vi "Drive_Strait.vi"(8 "Right MotorControlDevRef in":T1={"DeviceStatus"={"status"=FALSE, "code"=0, "source"=""}, "Type"=enum."PWM", "PWM"={"PWM Channel"=enum."Invalid", "DeadBand"={"Name"="", "maxPositivePwm"=0, "minPositivePwm"=0, "centerPwm"=0, "maxNegativePwm"=0, "minNegativePwm"=0, "angularRange"=0}}, "CAN"={"Device Number"=0, "SetOutput VI Ref"=variant(refnum<vi> refnum), "GetOutput VI Ref"=variant(refnum<vi> refnum), "Enable VI Ref"=variant(refnum<vi> refnum), "Disable VI Ref"=variant(refnum<vi> refnum), "Data"=variant}, "Invert"=FALSE}, 9 "Left MotorControlDevRef in":T1={"DeviceStatus"={"status"=FALSE, "code"=0, "source"=""}, "Type"=enum."PWM", "PWM"={"PWM Channel"=enum."Invalid", "DeadBand"={"Name"="", "maxPositivePwm"=0, "minPositivePwm"=0, "centerPwm"=0, "maxNegativePwm"=0, "minNegativePwm"=0, "angularRange"=0}}, "CAN"={"Device Number"=0, "SetOutput VI Ref"=variant(refnum<vi> refnum), "GetOutput VI Ref"=variant(refnum<vi> refnum), "Enable VI Ref"=variant(refnum<vi> refnum), "Disable VI Ref"=variant(refnum<vi> refnum), "Data"=variant}, "Invert"=FALSE}, 11 "Distance in":dbl format="%#_13g") -> (0 "Right MotorControlDevRef out":T1={"DeviceStatus"={"status"=FALSE, "code"=0, "source"=""}, "Type"=enum."PWM", "PWM"={"PWM Channel"=enum."Invalid", "DeadBand"={"Name"="", "maxPositivePwm"=0, "minPositivePwm"=0, "centerPwm"=0, "maxNegativePwm"=0, "minNegativePwm"=0, "angularRange"=0}}, "CAN"={"Device Number"=0, "SetOutput VI Ref"=variant(refnum<vi> refnum), "GetOutput VI Ref"=variant(refnum<vi> refnum), "Enable VI Ref"=variant(refnum<vi> refnum), "Disable VI Ref"=variant(refnum<vi> refnum), "Data"=variant}, "Invert"=FALSE}, 1 "Left MotorControlDevRef out":T1={"DeviceStatus"={"status"=FALSE, "code"=0, "source"=""}, "Type"=enum."PWM", "PWM"={"PWM Channel"=enum."Invalid", "DeadBand"={"Name"="", "maxPositivePwm"=0, "minPositivePwm"=0, "centerPwm"=0, "maxNegativePwm"=0, "minNegativePwm"=0, "angularRange"=0}}, "CAN"={"Device Number"=0, "SetOutput VI Ref"=variant(refnum<vi> refnum), "GetOutput VI Ref"=variant(refnum<vi> refnum), "Enable VI Ref"=variant(refnum<vi> refnum), "Disable VI Ref"=variant(refnum<vi> refnum), "Data"=variant}, "Invert"=FALSE}, 3 "Drive time out":u32)   [LabVIEW 2016]
uses:
  <vilib>/Rock Robotics/WPI/MotorControl/WPI_MotorControlDeviceRef.ctl
  <vilib>/Rock Robotics/WPI/MotorControl/WPI_MotorControlType.ctl
  <vilib>/Rock Robotics/SystemInterfaces/DIO/FPGA_DIOPWMChannel.ctl
  <vilib>/Rock Robotics/WPI/PWM/WPI_PWMDeadband.ctl
  <vilib>/Rock Robotics/WPI/ThirdParty/CanMotor/TalonSRX/WPI_CANTalonSRX_APIControlMode.ctl
panel:
  in  "Kp":dbl=0.375 format="%#_13g"
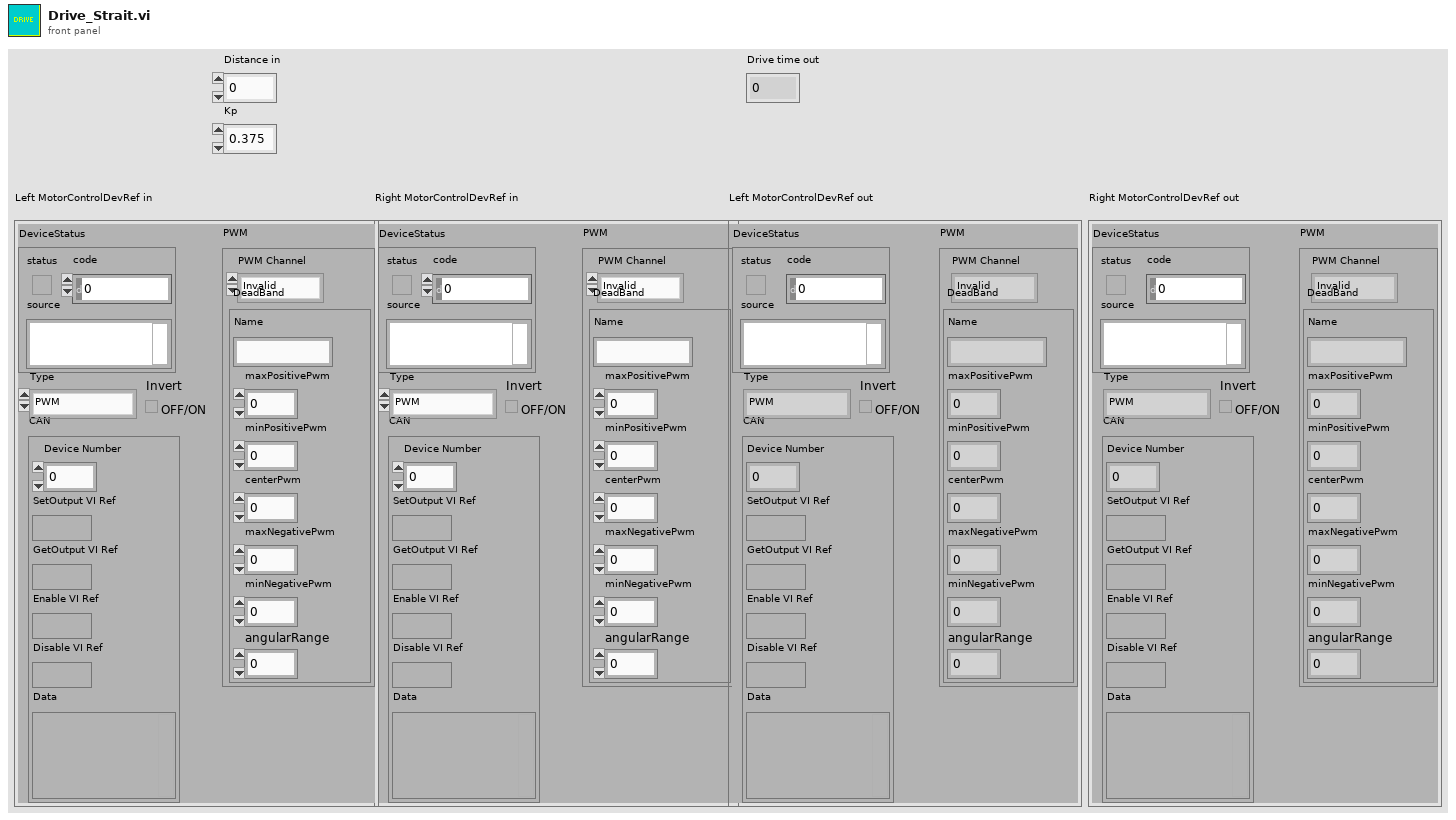
[diagram p1: front panel]
types:
  T1 = typedef "WPI_MotorControlDeviceRef.ctl" = cluster{"DeviceStatus":errorcluster, "Type":T2, "PWM":cluster{"PWM Channel":T3, "DeadBand":T4}, "CAN":cluster{"Device Number":u8, "SetOutput VI Ref":variant, "GetOutput VI Ref":variant, "Enable VI Ref":variant, "Disable VI Ref":variant, "Data":variant}, "Invert":bool}
  T2 = typedef "WPI_MotorControlType.ctl" = enum16{"PWM", "CAN"}
  T3 = typedef "FPGA_DIOPWMChannel.ctl" = enum8{"PWM 0", "PWM 1", "PWM 2", "PWM 3", "PWM 4", "PWM 5", "PWM 6", "PWM 7", "PWM 8", "PWM 9", "PWM MXP 0", "PWM MXP 1", "PWM MXP 2", "PWM MXP 3", "PWM MXP 4", "PWM MXP 5", "PWM MXP 6", "PWM MXP 7", "PWM MXP 8", "PWM MXP 9", "Invalid"}
  T4 = typedef "WPI_PWMDeadband.ctl" = cluster{"Name":string, "maxPositivePwm":i32, "minPositivePwm":i32, "centerPwm":i32, "maxNegativePwm":i32, "minNegativePwm":i32, "angularRange":u16}
  T5 = typedef "WPI_CANTalonSRX_APIControlMode.ctl" = enum8{"Percent VBus", "Speed", "Position", "Slave", "Unchanged / Invalid", "Voltage Compensation", "Current", "Motion Profile", "Motion Magic"}
  T6 = typedef "WPI_CANTalonSRX_GlobalStatus.ctl" = cluster{"Applied Throttle":dbl, "Module Enabled":bool, "CAN Error":errorcluster, "Closed Loop Error":dbl, "Forward Limit Switch Closed":bool, "Reverse Limit Switch Closed":bool, "Sensor Position":dbl, "Sensor Velocity":dbl, "Current":dbl, "Sticky Fault - Over Temp":bool, "Sticky Fault - Under Voltage":bool, "Sticky Fault - Forward Limit":bool, "Sticky Fault - Reverse Limit":bool, "Sticky Fault - Forward Soft Limit":bool, "Sticky Fault - Reverse Soft Limit":bool, "Brake is Enabled":bool, "Encoder Position":dbl, "Encoder Velocity":dbl, "Encoder Index Count":dbl, "Encoder A Pin State":bool, "Encoder B Pin State":bool, "Encoder Index Pin State":bool, "Analog In":dbl, "Analog In Velocity":dbl, "Temperature (C)":dbl, "Battery Voltage":dbl, "Control 5 Is Supported":bool, "Current Profile Slot Select":dbl, "Pos Div 8":bool, "Vel Div 4":bool, "Pulse Width Position":i32, "Pulse Width Velocity":i32, "Pulse Width Rise To Rise (us)":i32, "Pulse Width Rise To Fall (us)":i32, "Mot Prof Active Is Under Run":bool, "Mot Prof Active Has Under Run":bool, "Mot Prof Active Is Last":bool, "Mot Prof Active Velocity Only":bool, "Mot Prof Active Is Valid":bool, "Mot Prof Buffer Is Full":bool, "Mot Prof Active Profile Slot Select":i32, "Mot Prof NextID":i32, "Mot Prof Count":i32, "Mot Prof Active Velocity":dbl, "Mot Prof Active Position":dbl, "Mot Prof Output Enable":i32}
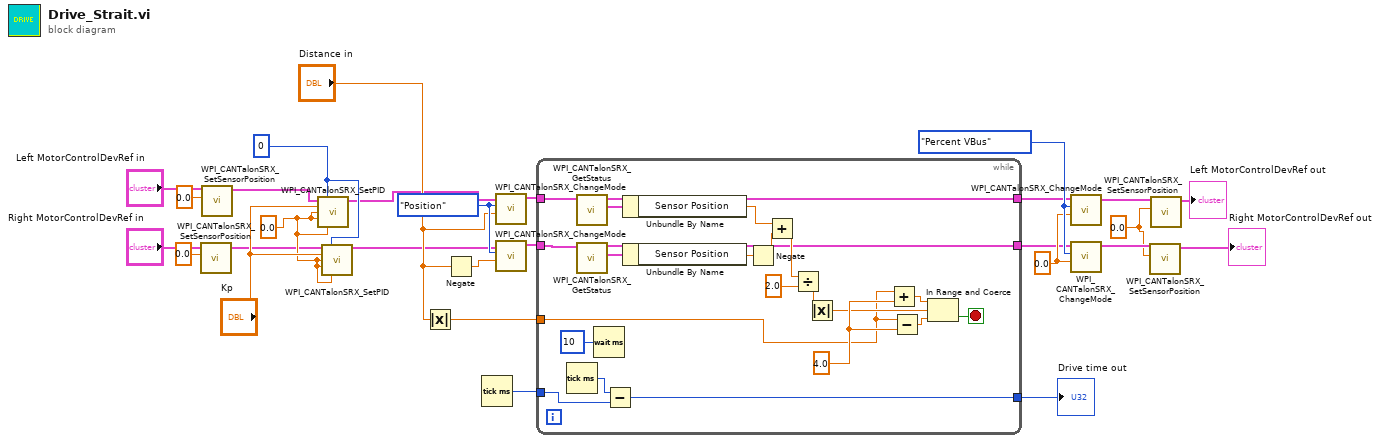
[diagram p0: block diagram]
diagram:
  w16 = WPI_CANTalonSRX_APIControlMode."Position" ("Control Mode")
  w3 = 0.0 ("New Sensor Position")
  w21 = 0.0
  w23 = u8 0
  w26 = 0.0
  w27 = WPI_CANTalonSRX_APIControlMode."Percent VBus" ("Control Mode")
  n1 = call <vilib>:"WPI_CANTalonSRX_SetSensorPosition.vi"("New Sensor Position"=0.0, "CAN Talon SRX Ref"="Right MotorControlDevRef in") -> ("CAN Talon SRX Ref"=w8:T1)  [unwired: 8 in, 1 out]
  n2 = call <vilib>:"WPI_CANTalonSRX_SetSensorPosition.vi"("New Sensor Position"=0.0, "CAN Talon SRX Ref"="Left MotorControlDevRef in") -> ("CAN Talon SRX Ref"=w9:T1)  [unwired: 8 in, 1 out]
  n3 = call <vilib>:"WPI_CANTalonSRX_SetPID.vi"("CAN Talon SRX Ref"=w9, "Parameter Slot"=w23, "P"="Kp", "I"=w21, "D"=w21, "F"=w21) -> ("CAN Talon SRX Ref"=w14:T1)  [unwired: 8 in, 1 out]
  n4 = call <vilib>:"WPI_CANTalonSRX_SetPID.vi"("CAN Talon SRX Ref"=w8, "Parameter Slot"=w23, "P"="Kp", "I"=w21, "D"=w21, "F"=w21) -> ("CAN Talon SRX Ref"=w12:T1)  [unwired: 8 in, 1 out]
  n5 = Absolute Value(x="Distance in") -> (abs(x)=w10:dbl)
  n6 = Negate(x="Distance in") -> (-x=w17:dbl)
  n7 = Tick Count (ms)() -> (millisecond timer value=w28:u32)
  n8 = call <vilib>:"WPI_CANTalonSRX_ChangeMode.vi"("Output"="Distance in", "Control Mode"=w16, "CAN Talon SRX Ref"=w14) -> ("CAN Talon SRX Ref"=w13:T1)  [unwired: 7 in, 1 out]
  n9 = call <vilib>:"WPI_CANTalonSRX_ChangeMode.vi"("Output"=w17, "Control Mode"=w16, "CAN Talon SRX Ref"=w12) -> ("CAN Talon SRX Ref"=w11:T1)  [unwired: 7 in, 1 out]
  n10 = while {
    tunnel: w13 -> [w47]
    tunnel: w11 -> [w46]
    tunnel: [w31] -> w7
    tunnel: [w30] -> w6
    tunnel: w28 -> [w50]
    tunnel: [w32] -> w18
    tunnel: w10 -> [w29]
    stop <- w38 stop-if-true
    w37 = 4.0
    n11 = Tick Count (ms)() -> (millisecond timer value=w49:u32)
    n12 = call <vilib>:"WPI_CANTalonSRX_GetStatus.vi"("CAN Talon SRX Ref"=w47) -> ("Talon SRX Status"=w45:T6, "CAN Talon SRX Ref"=w31:T1)  [unwired: 8 in, 1 out]
    n13 = call <vilib>:"WPI_CANTalonSRX_GetStatus.vi"("CAN Talon SRX Ref"=w46) -> ("Talon SRX Status"=w44:T6, "CAN Talon SRX Ref"=w30:T1)  [unwired: 8 in, 1 out]
    n14 = Wait (ms)(milliseconds to wait=u32 10) -> ()  [unwired: 1 out]
    n15 = Subtract(x=w49, y=w50) -> (x-y=w32:u32)
    n16 = Unbundle By Name(w45) -> ("Sensor Position"=w43:dbl)
    n17 = Unbundle By Name(w44) -> ("Sensor Position"=w42:dbl)
    n18 = Negate(x=w42) -> (-x=w34:dbl)
    n19 = Add(x=w43, y=w34) -> (x+y=w41:dbl)
    n20 = Divide(x=w41, y=2.0) -> (x/y=w39:dbl)
    n21 = Absolute Value(x=w39) -> (abs(x)=w33:dbl)
    n22 = Add(x=w29, y=w37) -> (x+y=w36:dbl)
    n23 = Subtract(x=w29, y=w37) -> (x-y=w35:dbl)
    n24 = In Range and Coerce(upper limit=w36, x=w33, lower limit=w35) -> (In Range?=w38:bool)  [unwired: 1 out]
  }
  "Drive time out" <- w18
  n25 = call <vilib>:"WPI_CANTalonSRX_ChangeMode.vi"("Output"=w26, "Control Mode"=w27, "CAN Talon SRX Ref"=w7) -> ("CAN Talon SRX Ref"=w5:T1)  [unwired: 7 in, 1 out]
  n26 = call <vilib>:"WPI_CANTalonSRX_ChangeMode.vi"("Output"=w26, "Control Mode"=w27, "CAN Talon SRX Ref"=w6) -> ("CAN Talon SRX Ref"=w4:T1)  [unwired: 7 in, 1 out]
  n27 = call <vilib>:"WPI_CANTalonSRX_SetSensorPosition.vi"("New Sensor Position"=w3, "CAN Talon SRX Ref"=w4) -> ("CAN Talon SRX Ref"=→"Right MotorControlDevRef out":T1)  [unwired: 8 in, 1 out]
  n28 = call <vilib>:"WPI_CANTalonSRX_SetSensorPosition.vi"("New Sensor Position"=w3, "CAN Talon SRX Ref"=w5) -> ("CAN Talon SRX Ref"=→"Left MotorControlDevRef out":T1)  [unwired: 8 in, 1 out]
